vi "EnableDisableFPControls.vi"(7 "Enable/Disable?":T1(ring)=enum."Disabled", 8 "error in (no error)":errorcluster, 11 "UI_Interaction_Manager in":refnum<class "UI_Interaction_Manager.lvclass">) -> (0 "error out":errorcluster, 3 "UI_Interaction_Manager out":refnum<class "UI_Interaction_Manager.lvclass">)   [LabVIEW 2011, in "UI_Interaction_Manager.lvclass"]
uses:
  UI_Interaction_Manager.lvclass
  UI_Interaction_Manager.lvclass/UI_Interaction_Manager.ctl
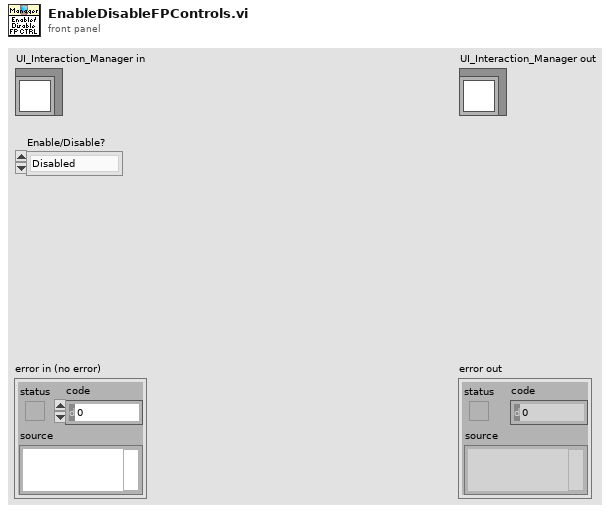
[diagram p1: front panel]
types:
  T1 = enum8{"Enabled", "Disabled", "Disabled and Grayed Out"}
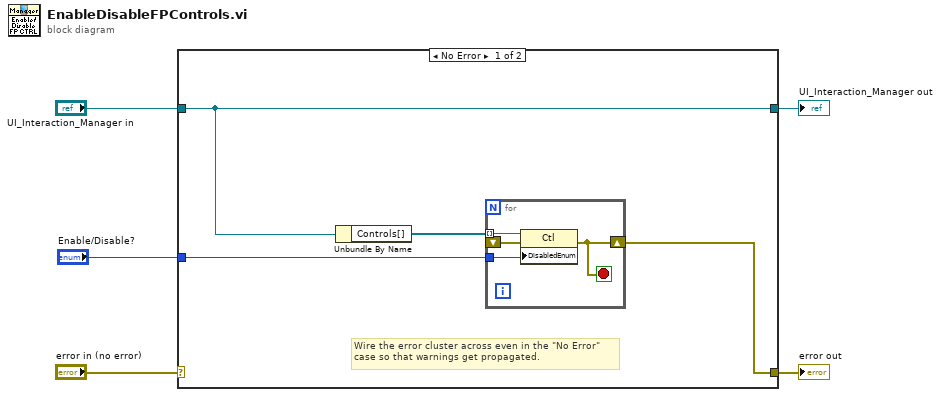
[diagram p0: block diagram]
diagram:
  n1 = case shown="No Error" "error in (no error)" {
    selector: "error in (no error)" -> [_ w15]
    tunnel: [w8 w15] -> w4
    tunnel: [w7 w14] -> w2
    tunnel: "UI_Interaction_Manager in" -> [w7 w14]
    tunnel: "Enable/Disable?" -> [w9 _]
    frame No Error {
      # "Wire the error cluster across even in the \"No Error\"\ncase so that warnings get propagated."
      n2 = Unbundle By Name(w7) -> ("Controls[]"=w6:refnum<vi>[])
      n3 = for {
        tunnel: w9 -> [w13]
        shift-right: [w11] -> w8
        shift-left: _ -> [w12]
        tunnel: w6 -> [w10] mode=indexing
        stop <- w11 stop-if-true
        n4 = property class="Ctl"(reference=w10, error in=w12, "DisabledEnum"=w13) -> (error out=w11:errorcluster)  [unwired: 1 out]
      }
    }
    frame Error {
    }
  }
  "error out" <- w4
  "UI_Interaction_Manager out" <- w2
